vi "BooleanProbe.vi"() -> ()   [LabVIEW 2010]
panel:
  out "Boolean":bool
  in  "Probe":bool
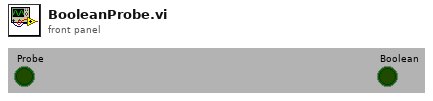
[diagram p1: front panel]
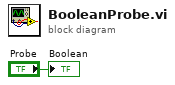
[diagram p0: block diagram]
diagram:
  "Boolean" <- "Probe"
